vi "emi_Anything Changed w init.vi"(7 "Anything":variant, 13 "Initial(void)":variant) -> (8 "changed":bool)   [LabVIEW 2010]
doc: "Compares any value with its previous value.\n\nOn first call, it reads the Initial input, and uses that as the previous value for comparison.\n\nUses variant, will except anything, note: Slow with large sets.\nDedicated type comparison will always be faster.\n\nreentrant Subroutine."
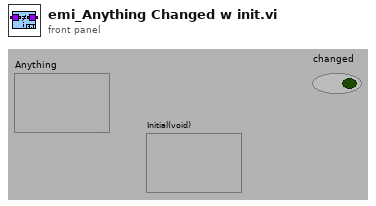
[diagram p1: front panel]
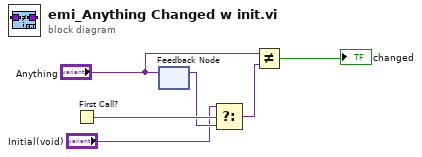
[diagram p0: block diagram]
diagram:
  n1 = First Call?() -> (First Call?: T/F=w6:bool)
  n2 = feedback-in #1("Anything") -> ()
  n3 = feedback #1() -> (w5:variant)  [unwired: 1 in]
  n4 = Select(t="Initial(void)", s=w6, f=w5) -> (s? t:f=w4:variant)
  n5 = Not Equal?(x="Anything", y=w4) -> (x != y?=→"changed":bool)
